vi "Color Sensor V3 Check Device ID.vi"(8 "error in (no error)":errorcluster, 11 "ColorSensorDevRef":T1={"I2CDevRef"={"DevStatus"={"status"=FALSE, "code"=0, "source"=""}, "Device Address"=0, "Handle"=0, "I2C Bus"=enum."Invalid"}} {"I2CDevRef"."Device Address" format="%.0x"}) -> (0 "error out":errorcluster, 3 "ColorSensorDevRef out":T1={"I2CDevRef"={"DevStatus"={"status"=FALSE, "code"=0, "source"=""}, "Device Address"=0, "Handle"=0, "I2C Bus"=enum."Invalid"}} {"I2CDevRef"."Device Address" format="%.0x"})   [LabVIEW 2023]
uses:
  Typedef/Color Sensor V3 DevRef.ctl
  <vilib>/Rock Robotics/WPI/I2C/WPI_I2CDevRef.ctl
  <vilib>/Rock Robotics/SystemInterfaces/i2clib/i2c_bus.ctl
  Typedef/Color Sensor V3 Registers.ctl
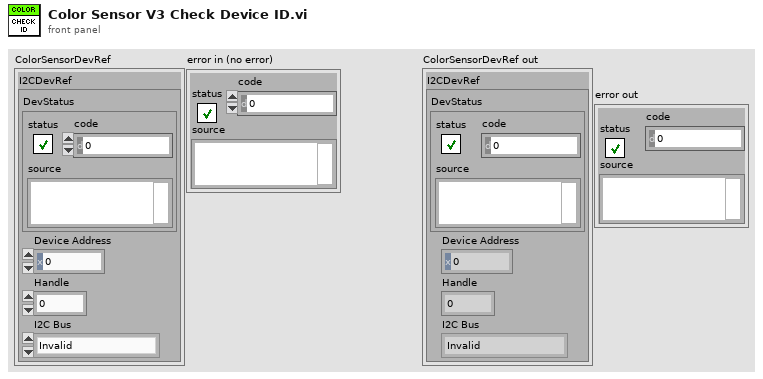
[diagram p1: front panel]
types:
  T1 = typedef "Color Sensor V3 DevRef.ctl" = cluster{"I2CDevRef":T2}
  T2 = typedef "WPI_I2CDevRef.ctl" = cluster{"DevStatus":errorcluster, "Device Address":u8, "Handle":i32, "I2C Bus":T3}
  T3 = typedef "i2c_bus.ctl" = enum16{"I2C On-Board", "I2C MXP", "Invalid"}
  T4 = typedef "Color Sensor V3 Registers.ctl" = enum16{"MainCtrl", "ProximitSensorLED", "ProximitySensorPulse", "ProximitySensorRate", "LightSensorMeasurementRate", "LightSensorGainRegister", "PartIDRegister", "MainStatus", "ProximityData", "ProximityData1", "InfraredData", "InfraredData1", "InfraredData2", "GreenData", "GreenData1", "GreenData2", "BlueData", "BlueData1", "BlueData2", "RedData", "RedData1", "RedData2"}
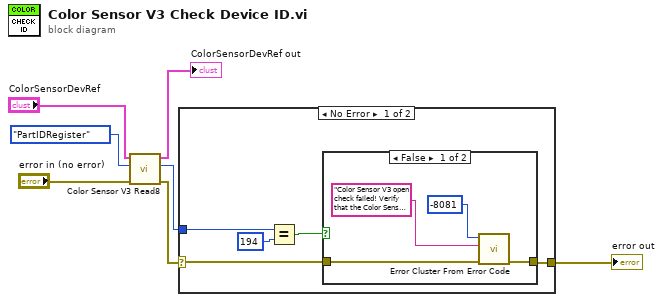
[diagram p0: block diagram]
diagram:
  n1 = call "Color Sensor V3 Read8.vi"("error in (no error)"="error in (no error)", "Registers"=Color_Sensor_V3_Registers."PartIDRegister", "ColorSensorDevRef"="ColorSensorDevRef") -> ("error out"=w3:errorcluster, "Data"=w2:u8, "ColorSensorDevRef out"=→"ColorSensorDevRef out":T1)  [unwired: 6 in]
  n2 = case shown="No Error" w3 {
    selector: w3 -> [w10 w18]
    tunnel: w2 -> [w12 _]
    tunnel: [w9 w18] -> w1
    frame No Error {
      n3 = Equal?(x=w12, y=u8 194) -> (x = y?=w8:bool)
      n4 = case shown="False" w8 {
        tunnel: w10 -> [w16 w17]
        tunnel: [w15 w17] -> w9
        frame False {
          n5 = call <vilib>:"Error Cluster From Error Code.vi"("error in (no error)"=w16, "error message (\"\")"="Color Sensor V3 open check failed! Verify that the Color Sensor V3 is plugged into this I2C port. " ("error message (\"\")"), "error code (0)"=-8081) -> ("error out"=w15:errorcluster)  [unwired: 6 in]
        }
        frame True {
        }
      }
    }
    frame Error {
    }
  }
  "error out" <- w1
